vi "Get LakeShore 370 Formated Parameters.vi"(0 "VISA Resource Name":refnum<visa-resource-name>, 1 "Initial String":string, 2 "Channels to scan (empty - don't use scanner option)":i32[](array[numeric]), 5 "error in (no error)":errorcluster) -> (7 "Parameters":string, 10 "data string":string, 13 "Data titles":string[](array[string])=["LS370_R (Ohm)"], 14 "VISA Resource Name Out":refnum<visa-resource-name>, 19 "error out":errorcluster)   [LabVIEW 2015]
uses:
  GPIB/VISA  Send Receive.vi
panel:
  in  "Offset":i32
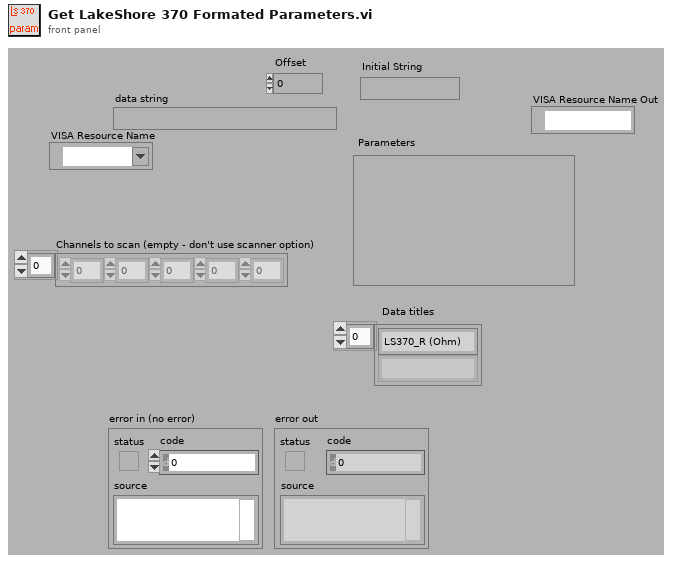
[diagram p1: front panel]
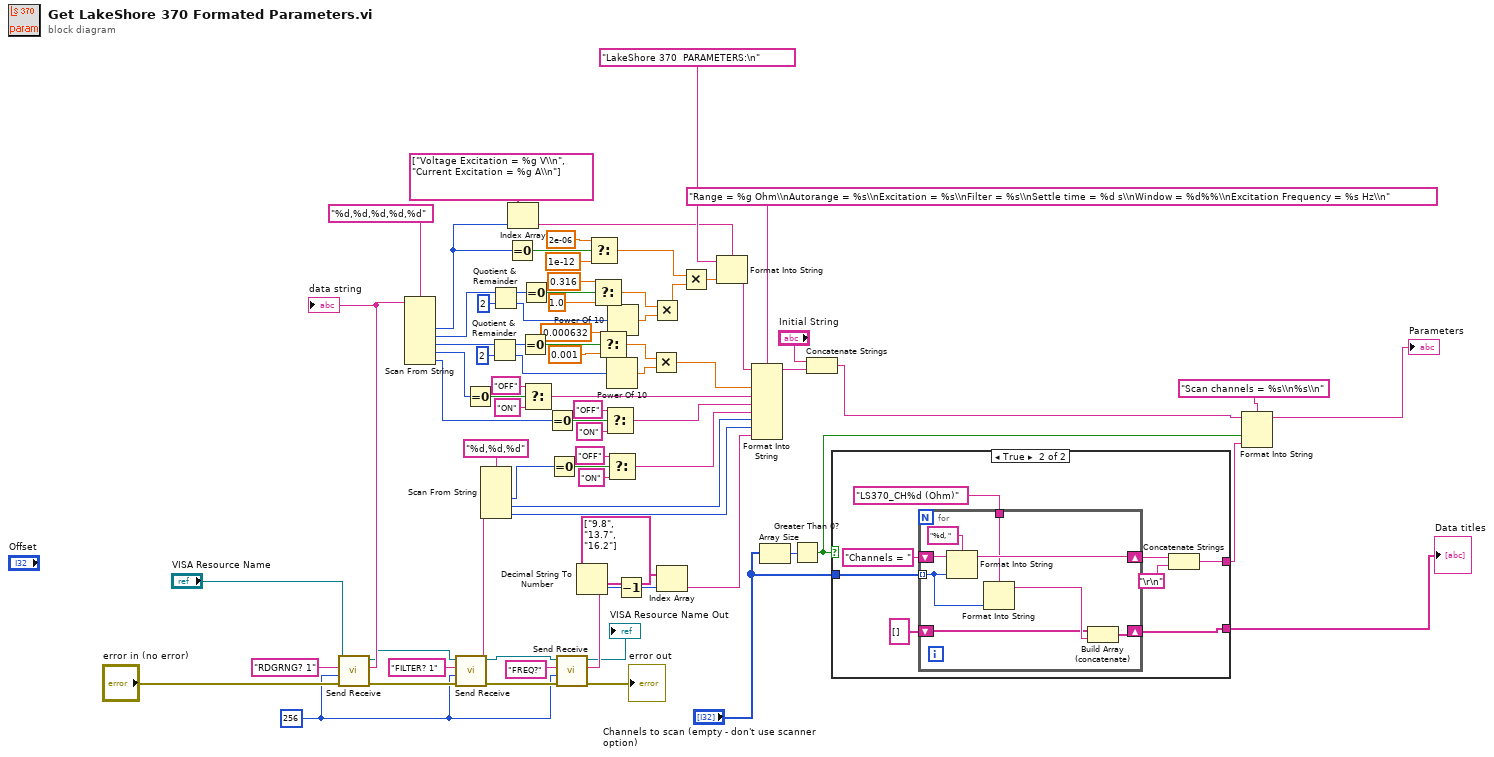
[diagram p0: block diagram]
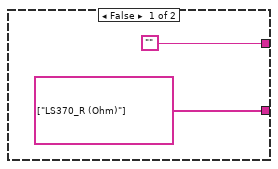
[diagram p2: hidden frame]
diagram:
  w21 = 256
  n1 = call-poly "Send Receive.vi"("error in (no error)"="error in (no error)", "Receive count"=w21, "data string in"="RDGRNG? 1", "VISA Resource Name"="VISA Resource Name") -> ("error out"=w34:errorcluster, "data string out"=w76:string, "VISA Resource Name Out"=w3:refnum<visa-resource-name>)  [unwired: 5 in]
  "data string" <- w76
  n2 = Scan From String(format string="%d,%d,%d,%d,%d", input string=w76) -> (output 1=w64:i32, output 2=w73:i32, output 3=w48:i32, output 4=w44:i32, output 5=w36:i32)  [unwired: 2 in, 8 out]
  n3 = call-poly "Send Receive.vi"("error in (no error)"=w34, "Receive count"=w21, "data string in"="FILTER? 1", "VISA Resource Name"=w3) -> ("error out"=w23:errorcluster, "data string out"=w31:string, "VISA Resource Name Out"=w2:refnum<visa-resource-name>)  [unwired: 5 in]
  n4 = Equal To 0?(x=w44) -> (x = 0?=w43:bool)
  n5 = Scan From String(format string="%d,%d,%d", input string=w31) -> (output 1=w27:i32, output 2=w24:i32, output 3=w25:i32)  [unwired: 2 in, 6 out]
  n6 = Quotient & Remainder(x=w48, y=2) -> (x-y*floor(x/y)=w55:i32, floor(x/y)=w51:i32)
  n7 = Quotient & Remainder(x=w73, y=2) -> (x-y*floor(x/y)=w71:i32, floor(x/y)=w63:i32)
  n8 = Equal To 0?(x=w64) -> (x = 0?=w67:bool)
  n9 = Index Array(array=string[] ["Voltage Excitation = %g V\\n", "Current Excitation = %g A\\n"], index=w64) -> (element=w58:string)
  n10 = Equal To 0?(x=w55) -> (x = 0?=w54:bool)
  n11 = Equal To 0?(x=w71) -> (x = 0?=w70:bool)
  n12 = Select(t="OFF", s=w43, f="ON") -> (s? t:f=w40:string)
  n13 = Equal To 0?(x=w36) -> (x = 0?=w39:bool)
  n14 = Equal To 0?(x=w27) -> (x = 0?=w30:bool)
  n15 = call-poly "Send Receive.vi"("error in (no error)"=w23, "Receive count"=w21, "data string in"="FREQ?", "VISA Resource Name"=w2) -> ("error out"=→"error out":errorcluster, "data string out"=w20:string, "VISA Resource Name Out"=→"VISA Resource Name Out":refnum<visa-resource-name>)  [unwired: 5 in]
  n16 = Decimal String To Number(string=w20) -> (number=w19:i32)  [unwired: 3 out]
  n17 = Select(t=2e-06, s=w67, f=1e-12) -> (s? t:f=w59:dbl)
  n18 = Select(t=0.316, s=w70, f=1.0) -> (s? t:f=w61:dbl)
  n19 = Select(t=0.000632, s=w54, f=0.001) -> (s? t:f=w49:dbl)
  n20 = Select(t="OFF", s=w39, f="ON") -> (s? t:f=w35:string)
  n21 = Power Of 10(x=w51) -> (10^x=w50:dbl)
  n22 = Select(t="OFF", s=w30, f="ON") -> (s? t:f=w26:string)
  n23 = Power Of 10(x=w63) -> (10^x=w62:dbl)
  n24 = Decrement(x=w19) -> (x-1=w17:i32)
  n25 = Multiply(x=w49, y=w50) -> (x*y=w46:dbl)
  n26 = Multiply(x=w61, y=w62) -> (x*y=w60:dbl)
  n27 = Index Array(array=string[] ["9.8", "13.7", "16.2"], index=w17) -> (element=w16:string)
  n28 = Multiply(x=w59, y=w60) -> (x*y=w57:dbl)
  n29 = Format Into String(format string=w58, initial string="LakeShore 370  PARAMETERS:\n", w57) -> (resulting string=w45:string)  [unwired: 1 in, 1 out]
  n30 = Format Into String(format string="Range = %g Ohm\\nAutorange = %s\\nExcitation = %s\\nFilter = %s\\nSettle time = %d s\\nWindow = %d%%\\nExcitation Frequency = %s Hz\\n", initial string=w45, w46, w40, w35, w26, w24, w25, w16) -> (resulting string=w15:string)  [unwired: 1 in, 1 out]
  n31 = Array Size(array="Channels to scan (empty - don't use scanner option)") -> (size(s)=w13:i32)
  n32 = Greater Than 0?(x=w13) -> (x > 0?=w11:bool)
  n33 = Concatenate Strings("Initial String", w15) -> (w7:string)
  n34 = case shown="True" w11 {
    tunnel: "Channels to scan (empty - don't use scanner option)" -> [_ w89]
    tunnel: ["" w85] -> w10
    tunnel: [string[] ["LS370_R (Ohm)"] ("Data titles") w82] -> w9
    frame False {
    }
    frame True {
      n35 = for {
        tunnel: w89 -> [w92] mode=indexing
        shift-right: [w95] -> w87
        shift-left: "Channels = " -> [w97]
        shift-right: [w93] -> w82
        shift-left: string[] [] -> [w90]
        tunnel: "LS370_CH%d (Ohm)" ("format string") -> [w94]
        n36 = Format Into String(format string="%d, ", initial string=w97, w92) -> (resulting string=w95:string)  [unwired: 1 in, 1 out]
        n37 = Format Into String(format string=w94, w92) -> (resulting string=w91:string)  [unwired: 2 in, 1 out]
        n38 = Build Array (concatenate)(w90, w91) -> (w93:string[])
      }
      n39 = Concatenate Strings(w87, "\r\n") -> (w85:string)
    }
  }
  "Data titles" <- w9
  n40 = Format Into String(format string="Scan channels = %s\\n%s\\n", initial string=w7, w11, w10) -> (resulting string=→"Parameters":string)  [unwired: 1 in, 1 out]
